vi "ReversedEngineering CreateNodes.vi"(1 "GraphRefToAddNodesTo":refnum<class "Graph.lvclass">, 2 "NodeClassInfoArray":T5[](array[typedef]), 3 "NodeClassInfo":T5, 4 "TypeDefs":T1[](array[typedef]), 5 "error in (no error)":errorcluster, 6 "Show Methods":bool=TRUE, 7 "graphics":refnum<class "Graphics.lvclass">, 8 "Show Attributes":bool=TRUE, 9 "grid":refnum<class "Grid.lvclass">, 11 "CreateTypeDefs":bool) -> (19 "error out":errorcluster)   [LabVIEW 2016]
uses:
  <resource>/Framework/Providers/Open_GDS/UML/ReversedEngineering/ReversedEngineering ClassInfoType.ctl
  <resource>/Framework/Providers/Open_GDS/UML/UMLEditor/UMLEditor_VisibilityType.ctl
  <resource>/Framework/Providers/Open_GDS/UML/ReversedEngineering/ReversedEngineering AttributeInfoType.ctl
  <resource>/Framework/Providers/Open_GDS/ClassProviders/Common/CommonVIs/CommonVIs_AttributeDataType.ctl
  <resource>/Framework/Providers/Open_GDS/UML/ReversedEngineering/ReversedEngineering_ClassDependencyDetailsType.ctl
  <resource>/Framework/Providers/Open_GDS/ClassProviders/Common/ScriptingFunctions/SubVIs/Scripting_ViDependencyType.ctl
  <resource>/Framework/Providers/Open_GDS/UML/Graph_class/Graph.lvclass
  <resource>/Framework/Providers/Open_GDS/UML/Graphics_class/Graphics.lvclass
  <resource>/Framework/Providers/Open_GDS/UML/Grid_class/Grid.lvclass
  <resource>/Framework/Providers/Open_GDS/UML/ReversedEngineering/ReversedEngineering TypeDefType.ctl
  <resource>/Framework/Providers/Open_GDS/UML/ClassNode_class/ExternalSetTypes.ctl
  <resource>/Framework/Providers/Open_GDS/UML/ClassNode_class/ClassNode.lvclass
  C:/Program Files (x86)/National Instruments/LabVIEW 2016/resource/Framework/Providers/Open_GDS/UML/RectangularNode_class/RectangularNode.lvclass
  C:/Program Files (x86)/National Instruments/LabVIEW 2016/resource/Framework/Providers/Open_GDS/UML/AbstractNode_class/AbstractNode.lvclass
  <resource>/Framework/Providers/Open_GDS/UML/AbstractNode_class/AbstractNode.lvclass
  <resource>/Framework/Providers/Open_GDS/UML/RectangularNode_class/RectangularNode.lvclass
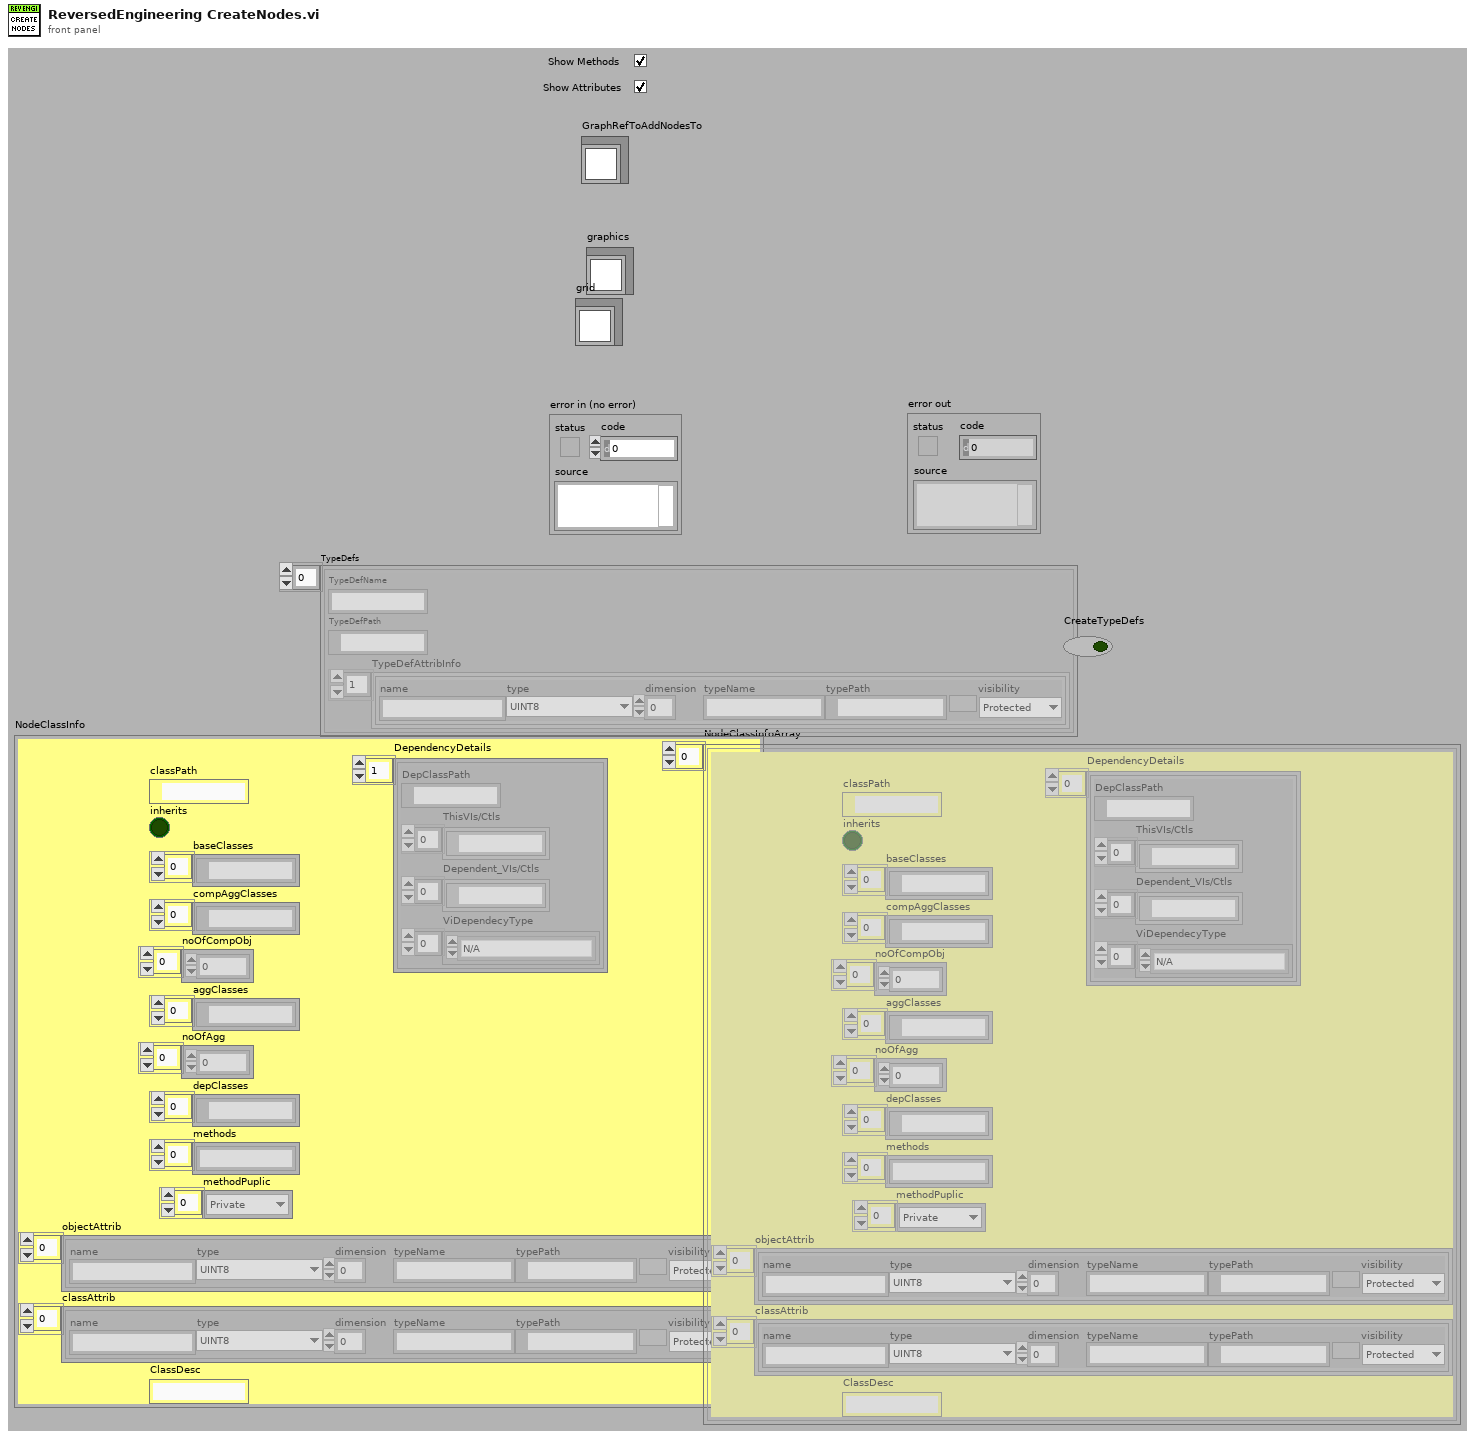
[diagram p1: front panel]
types:
  T1 = typedef "ReversedEngineering TypeDefType.ctl" = cluster{"TypeDefName":string, "TypeDefPath":path, "TypeDefAttribInfo":T2[]}
  T2 = typedef "ReversedEngineering AttributeInfoType.ctl" = cluster{"name":string, "type":T3, "dimension":i32, "typeName":string, "typePath":path, "visibility":T4}
  T3 = typedef "CommonVIs_AttributeDataType.ctl" = enum16{"UINT8", "INT8", "UINT16", "INT16", "UINT32", "INT32", "UINT64", "INT64", "SGL", "DBL", "EXT", "CSG", "CDB", "CXT", "TimeStamp", "STRING", "PATH", "BOOL", "ENUM", "RefNum", "VIRefNum", "LabVIEW Class", "Cluster", "Variant", "TypeDef", "Waveform", "LabVIEW Object", "Other", "void"}
  T4 = typedef "UMLEditor_VisibilityType.ctl" = enum16{"Public", "Private", "Protected"}
  T5 = typedef "ReversedEngineering ClassInfoType.ctl" = cluster{"classPath":path, "inherits":bool, "baseClasses":path[], "compAggClasses":path[], "noOfCompObj":i32[], "aggClasses":path[], "noOfAgg":i32[], "depClasses":path[], "methods":string[], "methodPuplic":T4[], "objectAttrib":T2[], "classAttrib":T2[], "ClassDesc":string, "DependencyDetails":T6[]}
  T6 = typedef "ReversedEngineering_ClassDependencyDetailsType.ctl" = cluster{"DepClassPath":path, "ThisVIs/Ctls":path[], "Dependent_VIs/Ctls":path[], "ViDependecyType":T7[]}
  T7 = typedef "Scripting_ViDependencyType.ctl" = enum16{"N/A", "Launches"}
  T8 = enum32{"None", "Stop", "Question", "Exclamation", "Information"}
  T9 = typedef "ClassNode.lvclass/ExternalSetTypes.ctl" = enum16{"Name", "Attributes", "Methods", "Position", "ShowMethods", "ShowAttributes", "ClassPath"}
  T10 = typedef "Rectangle Rectangle2D.ctl" = cluster{"x":dbl, "y":dbl, "width":dbl, "height":dbl}
  T11 = typedef "Point Point2D.ctl" = cluster{"x":dbl, "y":dbl}
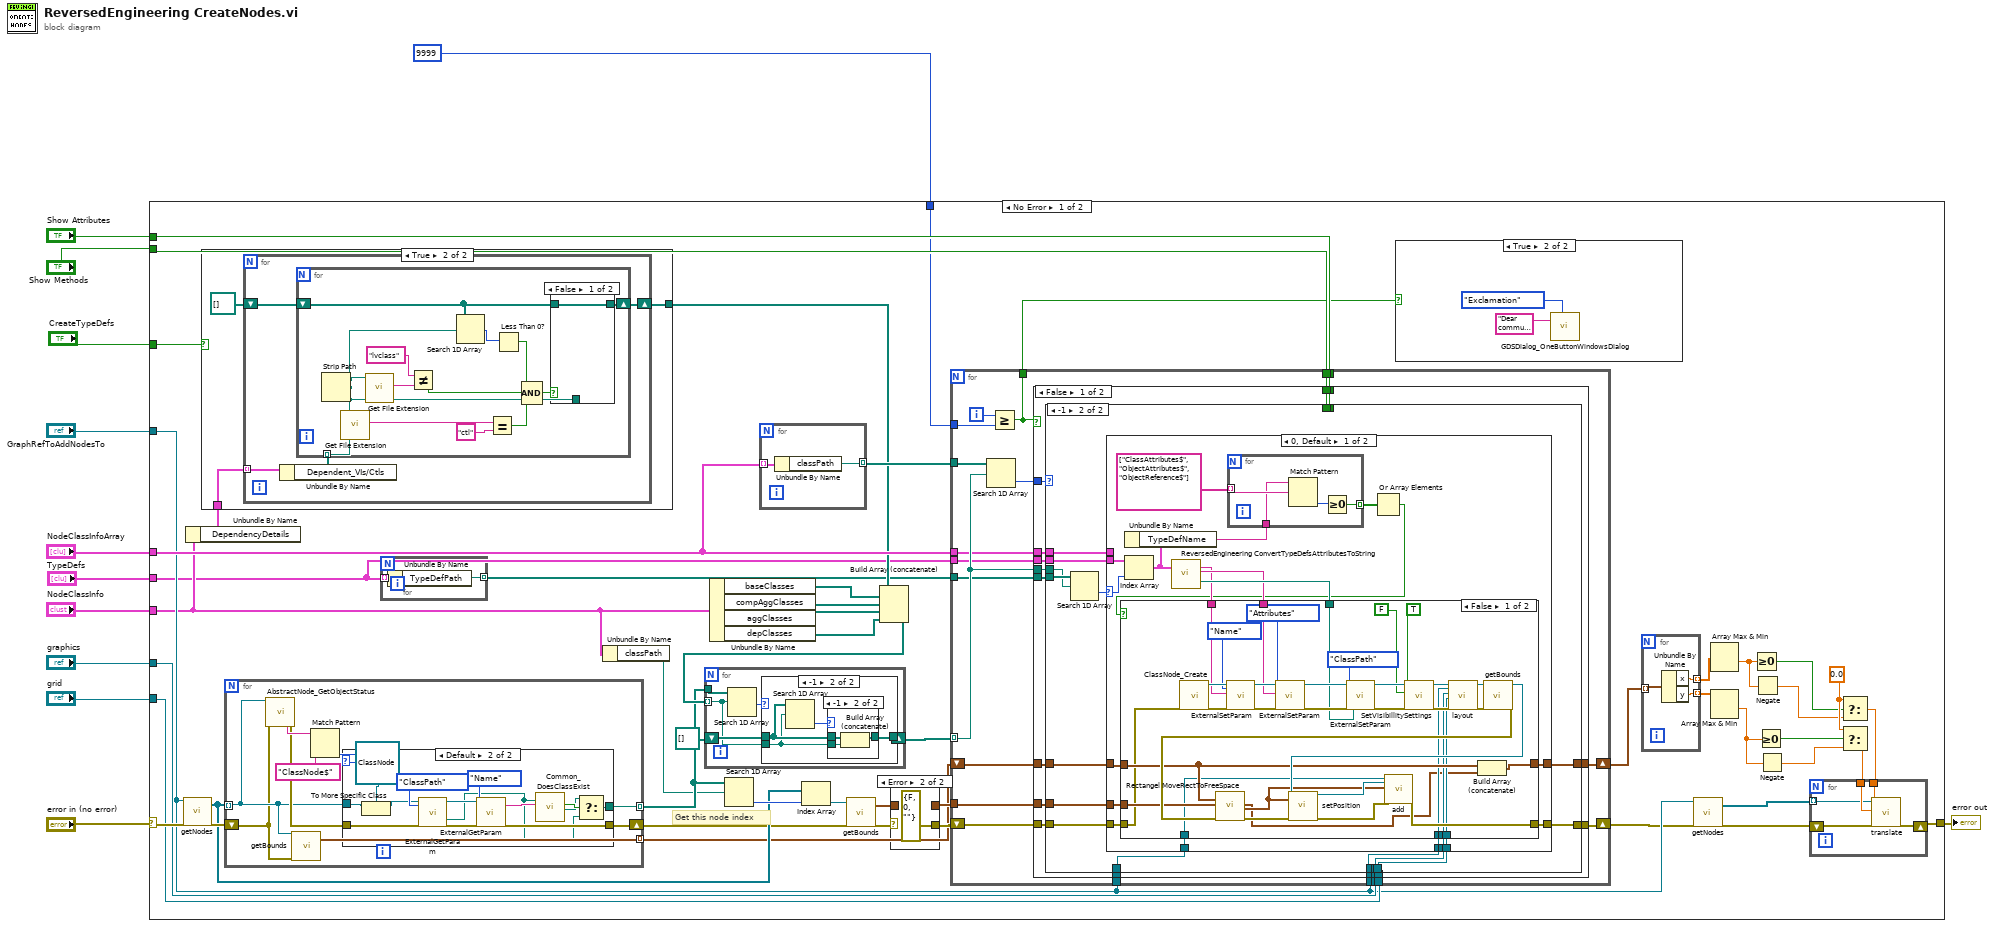
[diagram p0: block diagram]
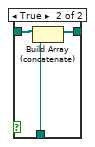
[diagram p4: hidden frame]
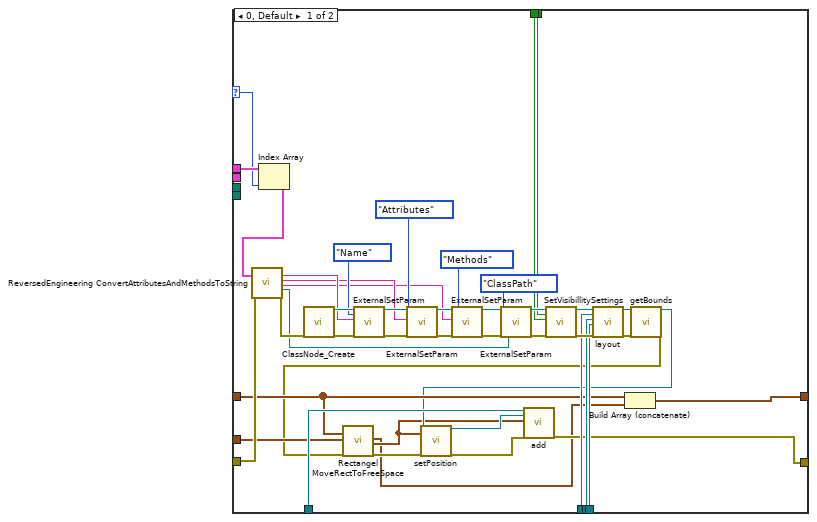
[diagram p8: hidden frame]
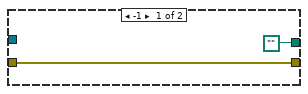
[diagram p12: hidden frame]
diagram:
  n1 = case shown="No Error" "error in (no error)" {
    selector: "error in (no error)" -> [w62 w302]
    tunnel: [w25 w302] -> w11
    tunnel: "Show Methods" -> [w43 _]
    tunnel: "NodeClassInfo" -> [w21 _]
    tunnel: "GraphRefToAddNodesTo" -> [w33 _]
    tunnel: "NodeClassInfoArray" -> [w55 _]
    tunnel: "Show Attributes" -> [w44 _]
    tunnel: "graphics" -> [w42 _]
    tunnel: "grid" -> [w41 _]
    tunnel: "CreateTypeDefs" -> [w17 _]
    tunnel: "TypeDefs" -> [w15 _]
    tunnel: i16 9999 -> [w14 _]
    frame No Error {
      w35 = 0.0 ("t")
      # "Get this node index"
      n2 = call-dynamic "getNodes.vi"("reference"=w33, "error in (no error)"=w62) -> ("nodes"=w50:refnum<class "AbstractNode.lvclass">[], "error out"=w61:errorcluster)  [unwired: 15 in, 1 out]
      n3 = Unbundle By Name(w21) -> ("DependencyDetails"=w20:T6[])
      n4 = case shown="True" w17 {
        tunnel: w20 -> [_ w69]
        tunnel: [_ w68] -> w18
        frame False {
        }
        frame True {
          n5 = for {
            tunnel: w69 -> [w73] mode=indexing
            shift-right: [w71] -> w68
            shift-left: path[] [] -> [w70]
            n6 = Unbundle By Name(w73) -> ("Dependent_VIs/Ctls"=w72:path[])
            n7 = for {
              tunnel: w72 -> [w79] mode=indexing
              shift-right: [w82] -> w71
              shift-left: w70 -> [w81]
              n8 = Strip Path(path=w79) -> (stripped path=w86:path)  [unwired: 1 out]
              n9 = call <vilib>:"Get File Extension.vi"("file"=w79) -> ("lowercase file extension"=w85:string)  [unwired: 1 in, 9 out]
              n10 = call <vilib>:"Get File Extension.vi"("file"=w86) -> ("lowercase file extension"=w77:string)  [unwired: 1 in, 9 out]
              n11 = Not Equal?(x="lvclass", y=w77) -> (x != y?=w74:bool)
              n12 = Search 1D Array(1D array=w81, element=w79) -> (index of element=w80:i32)  [unwired: 1 out]
              n13 = Equal?(x=w85, y="ctl") -> (x = y?=w75:bool)
              n14 = Less Than 0?(x=w80) -> (x < 0?=w78:bool)
              n15 = Compound Arithmetic op=AND(w78, w74, w75) -> (w83:bool)
              n16 = case shown="False" w83 {
                tunnel: [w87 w90] -> w82
                tunnel: w81 -> [w87 w89]
                tunnel: w79 -> [_ w88]
                frame False {
                }
                frame True {
                  n17 = Build Array (concatenate)(w89, w88) -> (w90:path[])
                }
              }
            }
          }
        }
      }
      n18 = for {
        tunnel: w50 -> [w279] mode=indexing
        shift-right: [w285] -> w49
        shift-left: w61 -> [w278]
        tunnel: [w284] -> w53 mode=indexing
        tunnel: [w277] -> w22 mode=indexing
        n19 = call <resource>:"AbstractNode_GetObjectStatus.vi"("reference in"=w279, "error in (no error)"=w278) -> ("Class name"=w283:string, "error out"=w282:errorcluster)  [unwired: 16 out]
        n20 = call-dynamic "getBounds.vi"("reference"=w279, "error in (no error)"=w278) -> ("bounds"=w277:T10)  [unwired: 15 in, 2 out]
        n21 = Match Pattern(string=w283, regular expression="ClassNode$") -> (offset past match=w280:i32)  [unwired: 4 out]
        n22 = case shown="Default" w280 {
          tunnel: w279 -> [_ w289]
          tunnel: w282 -> [w287 w296]
          tunnel: [w287 w295] -> w285
          tunnel: [path "" w291] -> w284
          frame -1 {
          }
          frame Default {
            n23 = To More Specific Class(target class=refnum<class "ClassNode.lvclass"> refnum ("reference"), reference=w289) -> (specific class reference=w288:refnum<class "ClassNode.lvclass">)  [unwired: 1 in, 1 out]
            n24 = call <resource>:"ExternalGetParam.vi"("reference"=w288, "setParameter"=ExternalSetTypes."ClassPath", "error in (no error)"=w296) -> ("reference out"=w300:refnum<class "ClassNode.lvclass">, "Path"=w293:path, "error out"=w299:errorcluster)  [unwired: 14 out]
            n25 = call <resource>:"ExternalGetParam.vi"("reference"=w300, "setParameter"=ExternalSetTypes."Name", "error in (no error)"=w299) -> ("string"=w297:string, "error out"=w295:errorcluster)  [unwired: 15 out]
            n26 = call <resource>:"Common_DoesClassExist.vi"("ClassPath"=w293, "ClassName"=w297) -> ("llb-class"=w294:bool, "llb/LvCLass-Path"=w292:path)  [unwired: 16 out]
            n27 = Select(t=w292, s=w294, f=w293) -> (s? t:f=w291:path)
          }
        }
      }
      n28 = for {
        tunnel: w15 -> [w66] mode=indexing
        tunnel: [w65] -> w16 mode=indexing
        n29 = Unbundle By Name(w66) -> ("TypeDefPath"=w65:path)
      }
      n30 = Unbundle By Name(w21) -> ("classPath"=w52:path)
      n31 = Unbundle By Name(w21) -> ("baseClasses"=w19:path[], "compAggClasses"=w60:path[], "aggClasses"=w59:path[], "depClasses"=w58:path[])
      n32 = Search 1D Array(1D array=w53, element=w52) -> (index of element=w51:i32)  [unwired: 1 out]
      n33 = for {
        tunnel: w55 -> [w117] mode=indexing
        tunnel: [w116] -> w54 mode=indexing
        n34 = Unbundle By Name(w117) -> ("classPath"=w116:path)
      }
      n35 = Index Array(array=w50, index=w51) -> (element=w48:refnum<class "AbstractNode.lvclass">)
      n36 = call-dynamic "getBounds.vi"("reference"=w48, "error in (no error)"=w49) -> ("bounds"=w45:T10, "error out"=w47:errorcluster)  [unwired: 15 in, 1 out]
      n37 = Build Array (concatenate)(w18, w19, w60, w59, w58) -> (w57:path[])
      n38 = for {
        tunnel: w57 -> [w102] mode=indexing
        tunnel: w53 -> [w106]
        shift-right: [w103] -> w56
        shift-left: path[] [] -> [w104]
        n39 = Search 1D Array(1D array=w106, element=w102) -> (index of element=w105:i32)  [unwired: 1 out]
        n40 = case shown="-1" w105 {
          tunnel: w104 -> [w107 w110]
          tunnel: [w107 w111] -> w103
          tunnel: w102 -> [_ w109]
          frame 0, Default {
          }
          frame -1 {
            n41 = Search 1D Array(1D array=w110, element=w109) -> (index of element=w108:i32)  [unwired: 1 out]
            n42 = case shown="-1" w108 {
              tunnel: w110 -> [w112 w115]
              tunnel: [w112 w114] -> w111
              tunnel: w109 -> [_ w113]
              frame 0, Default {
              }
              frame -1 {
                n43 = Build Array (concatenate)(w115, w113) -> (w114:path[])
              }
            }
          }
        }
      }
      n44 = case shown="Error" w47 {
        selector: w47 -> [w100 _]
        tunnel: [w100 errorcluster {"status"=FALSE, "code"=0, "source"=""} ("error in (no error)")] -> w46
        tunnel: w45 -> [w99 _]
        tunnel: [w99 _] -> w40
        frame No Error {
        }
        frame Error {
        }
      }
      n45 = for {
        tunnel: w54 -> [w137]
        tunnel: w56 -> [w135] mode=indexing
        shift-right: [w126] -> w26
        shift-left: w46 -> [w134]
        tunnel: w55 -> [w133]
        tunnel: w44 -> [w132]
        tunnel: w43 -> [w131]
        tunnel: w33 -> [w130]
        tunnel: w42 -> [w129]
        tunnel: w41 -> [w128]
        tunnel: w33 -> [w127]
        tunnel: w40 -> [w125]
        shift-right: [w123] -> w39
        shift-left: w22 -> [w124]
        tunnel: w16 -> [w122]
        tunnel: w15 -> [w121]
        tunnel: w14 -> [w119]
        tunnel: [w118] -> w13
        i -> [w120]
        n46 = Search 1D Array(1D array=w137, element=w135) -> (index of element=w136:i32)  [unwired: 1 out]
        n47 = Greater Or Equal?(x=w120, y=w119) -> (x >= y?=w118:bool)
        n48 = case shown="False" w118 {
          tunnel: w136 -> [w153 _]
          tunnel: w135 -> [w152 _]
          tunnel: w134 -> [w151 w275]
          tunnel: w133 -> [w150 _]
          tunnel: w132 -> [w149 _]
          tunnel: w131 -> [w148 _]
          tunnel: w130 -> [w147 _]
          tunnel: w129 -> [w146 _]
          tunnel: w128 -> [w145 _]
          tunnel: w127 -> [w144 _]
          tunnel: [w143 w275] -> w126
          tunnel: w125 -> [w142 _]
          tunnel: w124 -> [w141 w276]
          tunnel: [w140 w276] -> w123
          tunnel: w122 -> [w139 _]
          tunnel: w121 -> [w138 _]
          frame False {
            n49 = case shown="-1" w153 {
              selector: w153 -> [w179 _]
              tunnel: w152 -> [_ w210]
              tunnel: w151 -> [w181 w205]
              tunnel: w150 -> [w180 w204]
              tunnel: w149 -> [w171 _]
              tunnel: w148 -> [w170 _]
              tunnel: w147 -> [w169 w201]
              tunnel: w146 -> [w168 w200]
              tunnel: w145 -> [w167 w199]
              tunnel: w142 -> [w162 w203]
              tunnel: w144 -> [w166 w202]
              tunnel: [w165 w206] -> w143
              tunnel: w141 -> [w163 w208]
              tunnel: [w164 w207] -> w140
              tunnel: w139 -> [_ w211]
              tunnel: w138 -> [_ w198]
              frame 0, Default {
                n50 = Index Array(array=w180, index=w179) -> (element=w178:T5)
                n51 = call <resource>:"ReversedEngineering ConvertAttributesAndMethodsToString.vi"("classInfo"=w178, "error in (no error)"=w181) -> ("className"=w192:string, "attributes"=w189:string, "methods"=w185:string, "ClassPath"=w154:path, "error out"=w191:errorcluster)  [unwired: 13 out]
                n52 = call <resource>:"ClassNode_Create.vi"("error in (no error)"=w191) -> ("reference out"=w197:refnum<class "ClassNode.lvclass">, "error out"=w196:errorcluster)  [unwired: 1 in, 16 out]
                n53 = call-dynamic "ExternalSetParam.vi"("reference"=w197, "setParameter"=ExternalSetTypes."Name", "string"=w192, "error in (no error)"=w196) -> ("reference out"=w194:refnum<class "ClassNode.lvclass">, "error out"=w193:errorcluster)  [unwired: 14 in]
                n54 = call-dynamic "ExternalSetParam.vi"("reference"=w194, "setParameter"=ExternalSetTypes."Attributes", "string"=w189, "error in (no error)"=w193) -> ("reference out"=w187:refnum<class "ClassNode.lvclass">, "error out"=w188:errorcluster)  [unwired: 14 in]
                n55 = call-dynamic "ExternalSetParam.vi"("reference"=w187, "setParameter"=ExternalSetTypes."Methods", "string"=w185, "error in (no error)"=w188) -> ("reference out"=w183:refnum<class "ClassNode.lvclass">, "error out"=w184:errorcluster)  [unwired: 14 in]
                n56 = call-dynamic "ExternalSetParam.vi"("reference"=w183, "setParameter"=ExternalSetTypes."ClassPath", "error in (no error)"=w184, "ClassPath"=w154) -> ("reference out"=w172:refnum<class "ClassNode.lvclass">, "error out"=w173:errorcluster)  [unwired: 14 in]
                n57 = call <resource>:"SetVisibillitySettings.vi"("reference"=w172, "showAttribute"=w171, "showMethods"=w170, "error in (no error)"=w173) -> ("reference out"=w177:refnum<class "ClassNode.lvclass">, "error out"=w176:errorcluster)  [unwired: 14 out]
                n58 = call-dynamic "layout.vi"("reference"=w177, "graph"=w169, "graphics"=w168, "grid"=w167, "error in (no error)"=w176) -> ("reference out"=w175:refnum<class "ClassNode.lvclass">, "error out"=w174:errorcluster)  [unwired: 13 in]
                n59 = call-dynamic "getBounds.vi"("reference"=w175, "error in (no error)"=w174) -> ("reference out"=w159:refnum<class "ClassNode.lvclass">, "error out"=w161:errorcluster)  [unwired: 15 in, 1 out]
                n60 = call <resource>:"Rectangel MoveRectToFreeSpace.vi"("BoundsArray"=w163, "bounds"=w162, "error in (no error)"=w161) -> ("BoundsOut"=w155:T10, "point"=w157:T11, "error out"=w160:errorcluster)  [unwired: 1 in, 13 out]
                n61 = call <resource>:"setPosition.vi"("reference"=w159, "pos"=w157, "error in (no error)"=w160) -> ("reference out"=w158:refnum<class "ClassNode.lvclass">, "error out"=w156:errorcluster)  [unwired: 2 in, 13 out]
                n62 = call-dynamic "add.vi"("reference"=w166, "node"=w158, "point"=w157, "error in (no error)"=w156) -> ("error out"=w165:errorcluster)  [unwired: 13 in, 2 out]
                n63 = Build Array (concatenate)(w163, w155) -> (w164:T10[])
              }
              frame -1 {
                n64 = Search 1D Array(1D array=w211, element=w210) -> (index of element=w209:i32)  [unwired: 1 out]
                n65 = case shown="0, Default" w209 {
                  selector: w209 -> [w230 _]
                  tunnel: w208 -> [w228 w274]
                  tunnel: [w227 w274] -> w207
                  tunnel: [w226 w273] -> w206
                  tunnel: w205 -> [w220 w273]
                  tunnel: w204 -> [_ _]
                  tunnel: w203 -> [w229 _]
                  tunnel: w202 -> [w225 _]
                  tunnel: w201 -> [w224 _]
                  tunnel: w200 -> [w223 _]
                  tunnel: w199 -> [w222 _]
                  tunnel: w198 -> [w221 _]
                  frame 0, Default {
                    n66 = Index Array(array=w221, index=w230) -> (element=w214:T1)
                    n67 = Unbundle By Name(w214) -> ("TypeDefName"=w213:string)
                    n68 = call <resource>:"ReversedEngineering ConvertTypeDefsAttributesToString.vi"("TypeDef"=w214) -> ("className"=w217:string, "attributes"=w218:string, "ClassPath"=w219:path)  [unwired: 1 in, 15 out]
                    n69 = for {
                      tunnel: [w271] -> w216 mode=indexing
                      tunnel: string[] ["ClassAttributes$", "ObjectAttributes$", "ObjectReference$"] -> [w270] mode=indexing
                      tunnel: w213 -> [w269]
                      n70 = Match Pattern(string=w269, regular expression=w270) -> (offset past match=w272:i32)  [unwired: 4 out]
                      n71 = Greater Or Equal To 0?(x=w272) -> (x >= 0?=w271:bool)
                    }
                    n72 = Or Array Elements(Boolean array=w216) -> (logical OR=w212:bool)
                    n73 = case shown="False" w212 {
                      tunnel: w229 -> [w247 _]
                      tunnel: w228 -> [w246 w268]
                      tunnel: [w245 w268] -> w227
                      tunnel: [w244 w267] -> w226
                      tunnel: w225 -> [w243 _]
                      tunnel: w224 -> [w242 _]
                      tunnel: w223 -> [w241 _]
                      tunnel: w222 -> [w240 _]
                      tunnel: w220 -> [w235 w267]
                      tunnel: w219 -> [w234 _]
                      tunnel: w218 -> [w233 _]
                      tunnel: w217 -> [w232 _]
                      frame False {
                        n74 = call <resource>:"ClassNode_Create.vi"("error in (no error)"=w235) -> ("reference out"=w266:refnum<class "ClassNode.lvclass">, "error out"=w265:errorcluster)  [unwired: 1 in, 16 out]
                        n75 = call-dynamic "ExternalSetParam.vi"("reference"=w266, "setParameter"=ExternalSetTypes."Name", "string"=w232, "error in (no error)"=w265) -> ("reference out"=w263:refnum<class "ClassNode.lvclass">, "error out"=w262:errorcluster)  [unwired: 14 in]
                        n76 = call-dynamic "ExternalSetParam.vi"("reference"=w263, "setParameter"=ExternalSetTypes."Attributes", "string"=w233, "error in (no error)"=w262) -> ("reference out"=w238:refnum<class "ClassNode.lvclass">, "error out"=w239:errorcluster)  [unwired: 14 in]
                        n77 = call-dynamic "ExternalSetParam.vi"("reference"=w238, "setParameter"=ExternalSetTypes."ClassPath", "error in (no error)"=w239, "ClassPath"=w234) -> ("reference out"=w254:refnum<class "ClassNode.lvclass">, "error out"=w255:errorcluster)  [unwired: 14 in]
                        n78 = call <resource>:"SetVisibillitySettings.vi"("reference"=w254, "showAttribute"=TRUE, "showMethods"=FALSE, "error in (no error)"=w255) -> ("reference out"=w259:refnum<class "ClassNode.lvclass">, "error out"=w258:errorcluster)  [unwired: 14 out]
                        n79 = call-dynamic "layout.vi"("reference"=w259, "graph"=w242, "graphics"=w241, "grid"=w240, "error in (no error)"=w258) -> ("reference out"=w257:refnum<class "ClassNode.lvclass">, "error out"=w256:errorcluster)  [unwired: 13 in]
                        n80 = call-dynamic "getBounds.vi"("reference"=w257, "error in (no error)"=w256) -> ("reference out"=w251:refnum<class "ClassNode.lvclass">, "error out"=w253:errorcluster)  [unwired: 15 in, 1 out]
                        n81 = call <resource>:"Rectangel MoveRectToFreeSpace.vi"("BoundsArray"=w246, "bounds"=w247, "error in (no error)"=w253) -> ("BoundsOut"=w231:T10, "point"=w249:T11, "error out"=w252:errorcluster)  [unwired: 1 in, 13 out]
                        n82 = call <resource>:"setPosition.vi"("reference"=w251, "pos"=w249, "error in (no error)"=w252) -> ("reference out"=w250:refnum<class "ClassNode.lvclass">, "error out"=w248:errorcluster)  [unwired: 2 in, 13 out]
                        n83 = call-dynamic "add.vi"("reference"=w243, "node"=w250, "point"=w249, "error in (no error)"=w248) -> ("error out"=w244:errorcluster)  [unwired: 13 in, 2 out]
                        n84 = Build Array (concatenate)(w246, w231) -> (w245:T10[])
                      }
                      frame True {
                      }
                    }
                  }
                  frame -1 {
                  }
                }
              }
            }
          }
          frame True {
          }
        }
      }
      n85 = case shown="True" w13 {
        frame False {
        }
        frame True {
          n86 = call <resource>:"GDSDialog_OneButtonWindowsDialog.vi"("UserText"="Dear community user !\nYou have reached the limit of number of allowed classes for the community edition.\nYou have to upgrade to professional version to be able to have unlimited classes in the class diagram and the project." ("message"), "Icon"=T8."Exclamation") -> ()  [unwired: 8 in, 10 out]
        }
      }
      n87 = for {
        tunnel: w39 -> [w98] mode=indexing
        tunnel: [w97] -> w38 mode=indexing
        tunnel: [w96] -> w37 mode=indexing
        n88 = Unbundle By Name(w98) -> ("x"=w97:dbl, "y"=w96:dbl)
      }
      n89 = call-dynamic "getNodes.vi"("reference"=w33, "error in (no error)"=w26) -> ("nodes"=w24:refnum<class "AbstractNode.lvclass">[])  [unwired: 15 in, 2 out]
      n90 = Array Max & Min(array=w38) -> (min value=w31:dbl)  [unwired: 3 out]
      n91 = Array Max & Min(array=w37) -> (min value=w29:dbl)  [unwired: 3 out]
      n92 = Greater Or Equal To 0?(x=w31) -> (x >= 0?=w32:bool)
      n93 = Negate(x=w31) -> (-x=w30:dbl)
      n94 = Greater Or Equal To 0?(x=w29) -> (x >= 0?=w28:bool)
      n95 = Negate(x=w29) -> (-x=w27:dbl)
      n96 = Select(t=w35, s=w32, f=w30) -> (s? t:f=w36:dbl)
      n97 = Select(t=w35, s=w28, f=w27) -> (s? t:f=w34:dbl)
      n98 = for {
        tunnel: w36 -> [w95]
        tunnel: w34 -> [w94]
        shift-right: [w92] -> w25
        shift-left: w26 -> [w93]
        tunnel: w24 -> [w91] mode=indexing
        n99 = call-dynamic "translate.vi"("reference"=w91, "dx"=w95, "dy"=w94, "error in (no error)"=w93) -> ("error out"=w92:errorcluster)  [unwired: 14 in, 1 out]
      }
    }
    frame Error {
    }
  }
  "error out" <- w11
